vi "Publish Shutdown Complete.vi"(8 "error in (no error)":errorcluster, 11 "Process in":refnum<class "Process.lvclass">) -> (0 "error out":errorcluster, 3 "Process out":refnum<class "Process.lvclass">)   [LabVIEW 2019, in "TimingDRV Engine.lvlib" / "Process.lvclass"]
uses:
  Process.lvclass
  Process.lvclass/Process.ctl
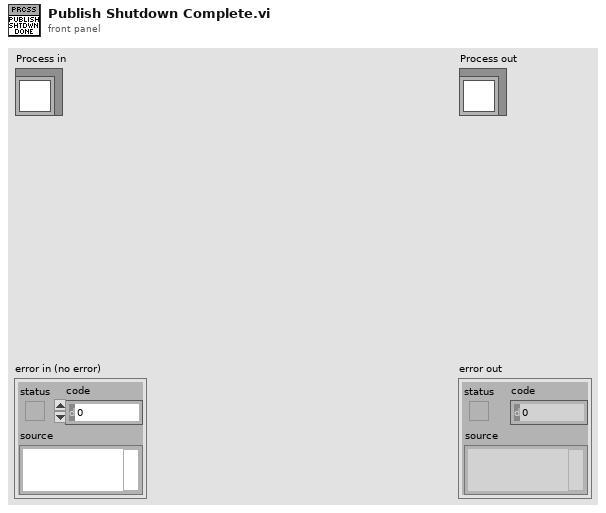
[diagram p1: front panel]
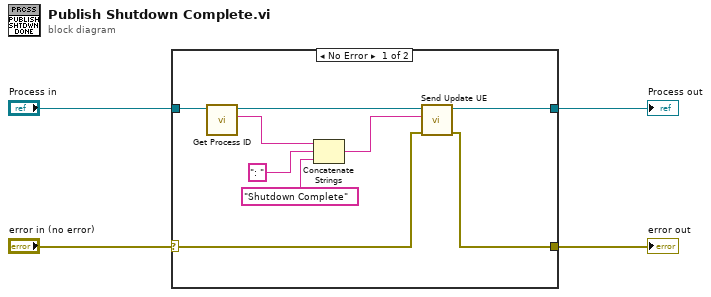
[diagram p0: block diagram]
diagram:
  n1 = case shown="No Error" "error in (no error)" {
    selector: "error in (no error)" -> [w6 w15]
    tunnel: [w5 w15] -> w3
    tunnel: [w7 w14] -> w1
    tunnel: "Process in" -> [w8 w14]
    frame No Error {
      n2 = call "Get Process ID.vi"("CD_Process in"=w8) -> ("Process ID"=w13:string, "CD_Process out"=w9:refnum<class "Process.lvclass">)  [unwired: 9 in]
      n3 = Concatenate Strings(w13, ": " ("string"), "Shutdown Complete" ("string")) -> (w10:string)
      n4 = call "Send Update UE.vi"("error in (no error)"=w6, "Update Message"=w10, "Process in"=w9) -> ("error out"=w5:errorcluster, "Process out"=w7:refnum<class "Process.lvclass">)  [unwired: 7 in]
    }
    frame Error {
    }
  }
  "error out" <- w3
  "Process out" <- w1
